vi "WLAN - Test - UTIL - Wait.vi"(8 "error in (no error)":errorcluster, 11 "Wait (ms)":u32) -> (0 "error out":errorcluster)   [LabVIEW 2011]
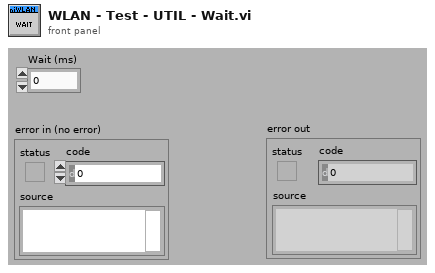
[diagram p1: front panel]
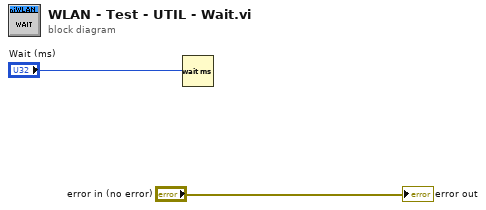
[diagram p0: block diagram]
diagram:
  n1 = Wait (ms)(milliseconds to wait="Wait (ms)") -> ()  [unwired: 1 out]
  "error out" <- "error in (no error)"
